vi "Create Error Cluster from Response Body.vi"(7 "AWS Core":refnum<class "HTTP Request.lvclass">, 8 "error in (no error)":errorcluster, 11 "Response body":string) -> (0 "error out":errorcluster, 3 "Is Throttled?":bool)   [LabVIEW 2015, in "NI_AWS_Core.lvlib" / "HTTP Request.lvclass"]
uses:
  HTTP Request.lvclass
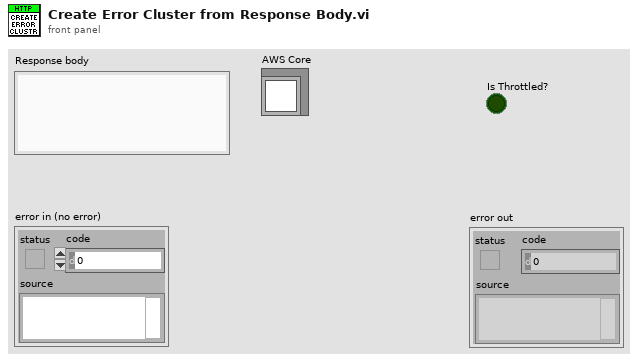
[diagram p1: front panel]
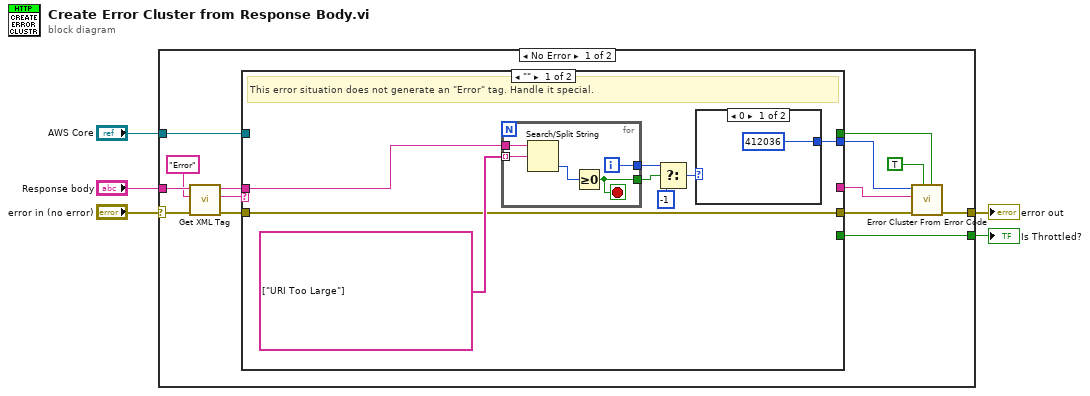
[diagram p0: block diagram]
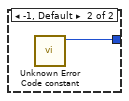
[diagram p2: hidden frame]
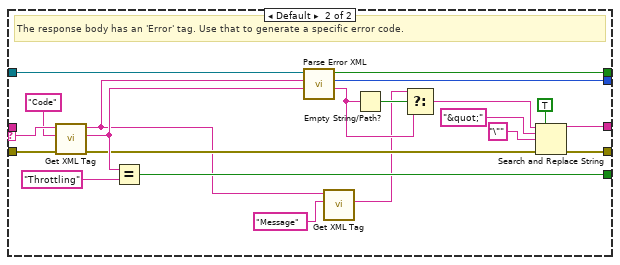
[diagram p3: hidden frame]
diagram:
  n1 = case shown="No Error" "error in (no error)" {
    selector: "error in (no error)" -> [w15 w56]
    tunnel: "Response body" -> [w19 _]
    tunnel: [w14 w56] -> w4
    tunnel: [w12 _] -> w2
    tunnel: "AWS Core" -> [w11 _]
    frame No Error {
      n2 = call "Get XML Tag.vi"("error in (no error)"=w15, "Tag name"="Error", "XML String in"=w19) -> ("error out"=w17:errorcluster, "Tag value"=w16:string, "XML String dup"=w6:string)  [unwired: 4 in, 2 out]
      n3 = case shown="\"\"" w16 {
        selector: w16 -> [_ w54]
        tunnel: w17 -> [w26 w55]
        tunnel: [_ w50] -> w12
        tunnel: w11 -> [_ w49]
        tunnel: [_ w48] -> w10
        tunnel: [w25 w47] -> w9
        tunnel: [w26 w43] -> w8
        tunnel: [_ w41] -> w7
        tunnel: w6 -> [w20 _]
        frame "" {
          # "This error situation does not generate an \"Error\" tag. Handle it special."
          n4 = for {
            tunnel: string[] ["URI Too Large"] -> [w30] mode=indexing
            tunnel: [w28] -> w24
            tunnel: [w31] -> w23
            tunnel: w20 -> [w29]
            i -> [w28]
            stop <- w31 stop-if-true
            n5 = Search/Split String(string=w29, search string/char (-)=w30) -> (offset of match=w32:i32)  [unwired: 1 in, 2 out]
            n6 = Greater Or Equal To 0?(x=w32) -> (x >= 0?=w31:bool)
          }
          n7 = Select(t=w24, s=w23, f=-1) -> (s? t:f=w22:i32)
          n8 = case shown="0" w22 {
            tunnel: [412036 w34] -> w25
            frame 0 {
            }
            frame -1, Default {
              n9 = call "Unknown Error Code constant.vi"() -> ("AWS Unknown Error Code value"=w34:i32)  [unwired: 11 in]
            }
          }
        }
        frame Default {
          # "The response body has an 'Error' tag. Use that to generate a specific error code."
          n10 = call "Get XML Tag.vi"("error in (no error)"=w55, "Tag name"="Code", "XML String in"=w54) -> ("error out"=w44:errorcluster, "Tag value"=w52:string, "XML String dup"=w39:string)  [unwired: 4 in, 2 out]
          n11 = Equal?(x=w52, y="Throttling") -> (x = y?=w50:bool)
          n12 = call-dynamic "Parse Error XML.vi"("Code Tag Value"=w52, "Error XML"=w39, "AWS Core"=w49) -> ("Error Description Override"=w37:string, "Error Code"=w47:i32, "Warning"=w48:bool)  [unwired: 6 in]
          n13 = call "Get XML Tag.vi"("Tag name"="Message", "XML String in"=w39) -> ("Tag value"=w35:string)  [unwired: 5 in, 4 out]
          n14 = Empty String/Path?(string/path=w37) -> (empty?=w38:bool)
          n15 = Select(t=w35, s=w38, f=w37) -> (s? t:f=w36:string)
          n16 = Search and Replace String(replace all?=TRUE ("replace all? (F)"), input string=w36, search string="&quot;", replace string="\"", error in=w44) -> (result string=w41:string, error out=w43:errorcluster)  [unwired: 3 in, 2 out]
        }
      }
      n17 = call <vilib>:"Error Cluster From Error Code.vi"("is warning? (False)"=w10, "show call chain? (False)"=TRUE, "error in (no error)"=w8, "error message (\"\")"=w7, "error code (0)"=w9) -> ("error out"=w14:errorcluster)  [unwired: 4 in]
    }
    frame Error {
    }
  }
  "error out" <- w4
  "Is Throttled?" <- w2
